vi "ModulationExample.vi"() -> ()   [LabVIEW 2020]
uses:
  <vilib>/Analysis/3filter.llb/Butterworth Filter (DBL).vi
  <vilib>/Analysis/NI_AALBase.lvlib
panel:
  out "Waveform Graph":waveform(dbl)[](graph)=[{"t0"=timestamp(0 s since 1904-01-01), "dt"=0.0001, "Y"=array[10000 elements]}, {"t0"=timestamp(0 s since 1904-01-01), "dt"=0.0001, "Y"=array[10000 elements]}]
  in  "Filter Control":cluster{"Fc":dbl, "Order":i32}={"Fc"=100.0, "Order"=2} {"Fc" format="%.2p"}
  in  "Sampling Info":cluster{"Fs":dbl, "#s":dbl}={"Fs"=10000.0, "#s"=10000.0} {"Fs" format="%.2p"}
  in  "Carrier Frequency (Hz)":dbl=1000.0
  in  "Messenger #1 Type":enum16{"Sine", "Sawtooth", "Square", "Triangle"}(ring)
  in  "Messenger #2 Type":enum16{"Sine", "Sawtooth", "Square", "Triangle"}(ring)=enum."Sawtooth"
  in  "Messenger #2 Control":T1={"Frequency (Hz)"=10.0, "Amplitude (V)"=1.0, "Phase (°)"=0.0}
  in  "Messenger #1 Control":T1={"Frequency (Hz)"=10.0, "Amplitude (V)"=1.0, "Phase (°)"=0.0}
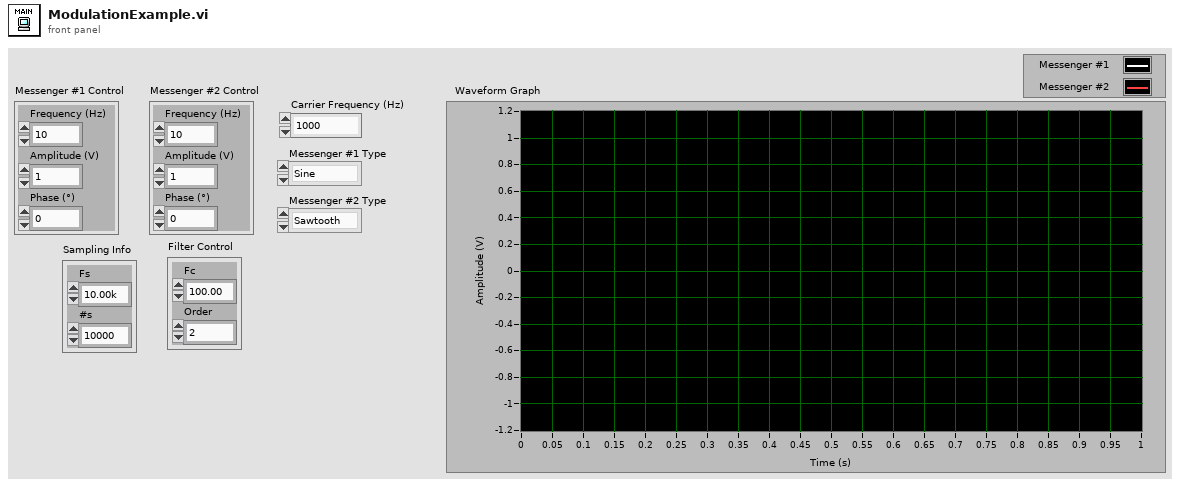
[diagram p1: front panel]
types:
  T1 = cluster{"Frequency (Hz)":dbl, "Amplitude (V)":dbl, "Phase (°)":dbl}
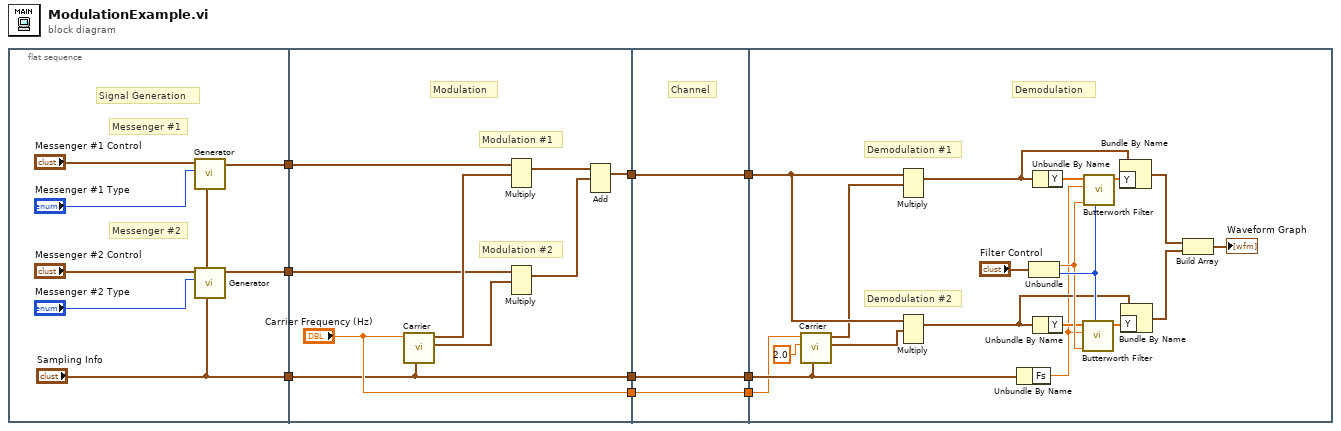
[diagram p0: block diagram]
diagram:
  n1 = flat-sequence {
    tunnel: [w14] -> w9
    tunnel: ["Sampling Info"] -> w8
    tunnel: [w12] -> w1
    tunnel: w9 -> [w24]
    tunnel: w8 -> [w18]
    tunnel: [w22] -> w7
    tunnel: ["Carrier Frequency (Hz)"] -> w4
    tunnel: [w18] -> w2
    tunnel: w1 -> [w17]
    tunnel: w7 -> [w28]
    tunnel: [w28] -> w6
    tunnel: [w27] -> w5
    tunnel: w4 -> [w27]
    tunnel: [w26] -> w3
    tunnel: w2 -> [w26]
    tunnel: w6 -> [w47]
    tunnel: w5 -> [w30]
    tunnel: w3 -> [w31]
    frame #0 {
      # "Messenger #2"
      # "Signal Generation"
      # "Messenger #1"
      n2 = call "Generator.vi"("Sampling Info"="Sampling Info", "Messenger Type (Sine)"="Messenger #1 Type", "Messenger Control"="Messenger #1 Control") -> ("Signal Out"=w14:waveform(dbl))  [unwired: 7 in, 1 out]
      n3 = call "Generator.vi"("Sampling Info"="Sampling Info", "Messenger Type (Sine)"="Messenger #2 Type", "Messenger Control"="Messenger #2 Control") -> ("Signal Out"=w12:waveform(dbl))  [unwired: 7 in, 1 out]
    }
    frame #1 {
      # "Modulation"
      # "Modulation #2"
      # "Modulation #1"
      n4 = call "Carrier.vi"("Sampling Info (10kS/s)"=w18, "Carrier Frequency (1kHz)"="Carrier Frequency (Hz)") -> ("Shifted Carrier"=w19:waveform(dbl), "Carrier"=w20:waveform(dbl))  [unwired: 7 in, 1 out]
      n5 = Multiply(1:w20, 2:w24) -> (0:w23:waveform(dbl))  [unwired: 1 in, 1 out]
      n6 = Multiply(1:w19, 2:w17) -> (0:w25:waveform(dbl))  [unwired: 1 in, 1 out]
      n7 = Add(1:w25, 2:w23) -> (0:w22:waveform(dbl))  [unwired: 1 in, 1 out]
    }
    frame #2 {
      # "Channel"
    }
    frame #3 {
      # "Demodulation #2"
      # "Demodulation #1"
      # "Demodulation"
      n8 = call "Carrier.vi"("Sampling Info (10kS/s)"=w31, "Carrier Amplitude (1V)"=2.0, "Carrier Frequency (1kHz)"=w30) -> ("Shifted Carrier"=w32:waveform(dbl), "Carrier"=w33:waveform(dbl))  [unwired: 6 in, 1 out]
      n9 = Multiply(1:w33, 2:w47) -> (0:w39:waveform(dbl))  [unwired: 1 in, 1 out]
      n10 = Multiply(1:w32, 2:w47) -> (0:w38:waveform(dbl))  [unwired: 1 in, 1 out]
      n11 = Unbundle By Name(w31) -> ("Fs"=w34:dbl)
      n12 = Unbundle("Filter Control") -> ("Fc"=w44:dbl, "Order"=w45:i32)
      n13 = Unbundle By Name(w39) -> ("Y"=w43:dbl[])
      n14 = Unbundle By Name(w38) -> ("Y"=w42:dbl[])
      n15 = call-poly <vilib>:"Butterworth Filter.vi"("order"=w45, "low cutoff freq: fl"=w44, "sampling freq: fs"=w34, "X"=w42) -> ("Filtered X"=w41:dbl[])  [unwired: 4 in, 1 out]
      n16 = call-poly <vilib>:"Butterworth Filter.vi"("order"=w45, "low cutoff freq: fl"=w44, "sampling freq: fs"=w34, "X"=w43) -> ("Filtered X"=w40:dbl[])  [unwired: 4 in, 1 out]
      n17 = Bundle By Name(cluster=w39, "Y"=w40) -> (w37:waveform(dbl))
      n18 = Bundle By Name(cluster=w38, "Y"=w41) -> (w36:waveform(dbl))
      n19 = Build Array(w37, w36) -> (→"Waveform Graph":waveform(dbl)[])
    }
  }
